vi "STM_Client.vi"() -> ()   [LabVIEW 2019, in "RemoteControl.STM.lvclass"]
uses:
  RemoteControl.STM.lvclass
  <vilib>/NI/STM/SubVIs/MetaDataElement.ctl
  <vilib>/NI/STM/TCP/Read Meta Data (TCP Ref).vi
  <vilib>/NI/STM/TCP/Get Connection Reference (TCP).vi
  <vilib>/NI/STM/TCP/Read Meta Data (TCP Clst).vi
  <userlib>/_OpenG.lib/numeric/numeric.llb/Random Number Within Range - I32__ogtk.vi
  <vilib>/NI/STM/TCP/Write Message (TCP).vi
  <vilib>/NI/STM/TCP/Read Message (TCP).vi
  <userlib>/_OpenG.lib/error/error.llb/Filter Error Codes (Array)__ogtk.vi
  <vilib>/NI/STM/NI STM.lvlib
panel:
  out "Numeric 2":i32
  out "Numeric":i32
  out "messsages/s":dbl
  in  "stop":bool
  out "reponse command":string
  out "response data":string
  out "Command":string
  out "duration ms":u32
  in  "remote address":string
  out "meta data\n(available commands)":T1[](array[typedef])
  out "error out":errorcluster
  # "CLIENT (API)"
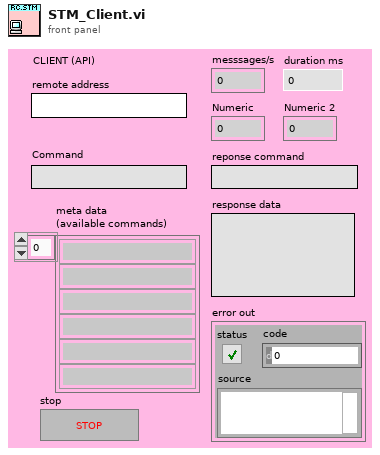
[diagram p1: front panel]
types:
  T1 = typedef "NI STM.lvlib/MetaDataElement.ctl" = string
  T2 = typedef "NI STM.lvlib/TCP Connection Info.ctl" = cluster{"connection ID":refnum<k5>, "meta data":T1[]}
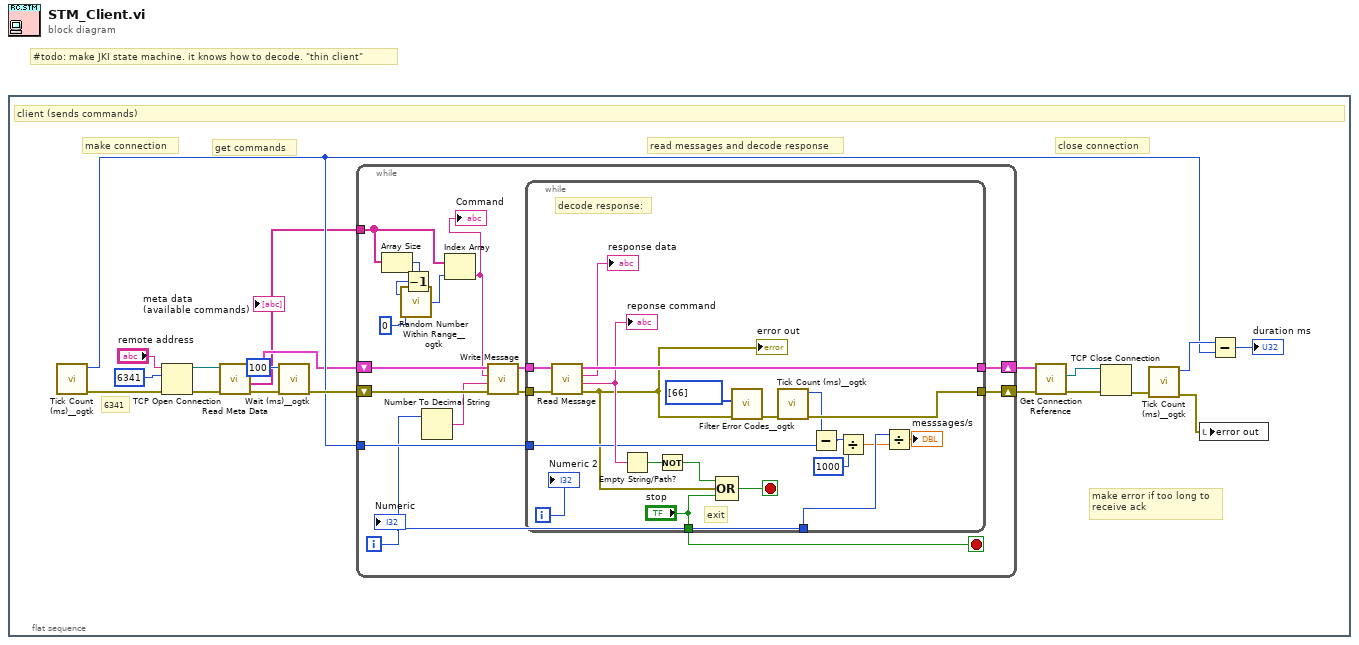
[diagram p0: block diagram]
diagram:
  # "#todo: make JKI state machine. it knows how to decode. \"thin client\""
  n1 = flat-sequence {
    frame #0 {
      # "close connection"
      # "read messages and decode response"
      # "get commands"
      # "make connection"
      # "6341"
      # "make error if too long to\nreceive ack"
      # "client (sends commands)"
      n2 = call <userlib>:"Tick Count (ms)__ogtk.vi"() -> ("error out"=w14:errorcluster, "millisecond timer value"=w4:u32)  [unwired: 10 in]
      n3 = TCP Open Connection(address="remote address", remote port or service name=u16 6341, error in (no error)=w14) -> (connection ID=w18:refnum<k5>, error out=w19:errorcluster)  [unwired: 2 in]
      n4 = call-poly <vilib>:"Read Meta Data.vi"("error in"=w19, "connection ID"=w18) -> ("error out"=w7:errorcluster, "meta data"=w2:T1[], "connection info out"=w3:T2)  [unwired: 7 in]
      "meta data\n(available commands)" <- w2
      n5 = call <userlib>:"Wait (ms)__ogtk.vi"("error in (no error)"=w7, "milliseconds to wait"=u32 100) -> ("error out"=w6:errorcluster)  [unwired: 8 in, 1 out]
      n6 = while {
        shift-right: [w33] -> w13
        shift-left: w6 -> [w28]
        shift-right: [w32] -> w12
        shift-left: w3 -> [w31]
        tunnel: w4 -> [w29]
        tunnel: w2 -> [w25]
        i -> [w21]
        stop <- w30 stop-if-true
        n7 = Array Size(array=w25) -> (size(s)=w26:i32)
        n8 = Decrement(x=w26) -> (x-1=w22:i32)
        n9 = call-poly <userlib>:"Random Number Within Range__ogtk.vi"("High"=w22, "Low"=0) -> ("Random Number"=w23:i32)  [unwired: 3 in]
        n10 = Number To Decimal String(number=w21) -> (decimal integer string=w20:string)  [unwired: 1 in]
        n11 = Index Array(array=w25, index=w23) -> (element=w24:T1)
        "Command" <- w24
        n12 = call-poly <vilib>:"Write Message.vi"("error in"=w28, "data"=w20, "name"=w24, "connection info in"=w31) -> ("error out"=w35:errorcluster, "connection info out"=w34:T2)  [unwired: 6 in]
        n13 = while {
          tunnel: w35 -> [w56]
          tunnel: w34 -> [w55]
          tunnel: [w45] -> w33
          tunnel: [w54] -> w32
          tunnel: ["stop"] -> w30
          tunnel: w29 -> [w43]
          tunnel: w21 -> [w40]
          i -> [w37]
          stop <- w53 stop-if-true
          # "decode response:"
          # "exit"
          n14 = call-poly <vilib>:"Read Message.vi"("error in"=w56, "connection info in"=w55) -> ("error out"=w36:errorcluster, "name"=w50:T1, "data string"=→"response data":string, "connection info out"=w54:T2)  [unwired: 2 in, 4 out]
          "reponse command" <- w50
          "error out" <- w36
          n15 = Empty String/Path?(string/path=w50) -> (empty?=w49:bool)
          n16 = Not(x=w49) -> (.not. x?=w48:bool)
          n17 = Compound Arithmetic op=OR(w48, w36, "stop") -> (w53:bool)
          n18 = call-poly <userlib>:"Filter Error Codes__ogtk.vi"("Error In"=w36, "Error Codes to Filter"=i32[] [66]) -> ("Error Out"=w46:errorcluster)  [unwired: 7 in, 2 out]
          n19 = call <userlib>:"Tick Count (ms)__ogtk.vi"("error in (no error)"=w46) -> ("error out"=w45:errorcluster, "millisecond timer value"=w44:u32)  [unwired: 9 in]
          n20 = Subtract(x=w44, y=w43) -> (x-y=w42:u32)
          n21 = Divide(x=w42, y=u32 1000) -> (x/y=w39:dbl)
          n22 = Divide(x=w40, y=w39) -> (x/y=→"messsages/s":dbl)
          "Numeric 2" <- w37
        }
        "Numeric" <- w21
      }
      n23 = call-poly <vilib>:"Get Connection Reference.vi"("error in"=w13, "connection info in"=w12) -> ("error out"=w16:errorcluster, "connection ID out"=w15:refnum<k5>)  [unwired: 7 in, 1 out]
      n24 = TCP Close Connection(connection ID=w15, error in (no error)=w16) -> (error out=w11:errorcluster)  [unwired: 1 in, 1 out]
      n25 = call <userlib>:"Tick Count (ms)__ogtk.vi"("error in (no error)"=w11) -> ("error out"=w1:errorcluster, "millisecond timer value"=w9:u32)  [unwired: 9 in]
      n26 = local write "error out"(w1) -> ()
      n27 = Subtract(x=w9, y=w4) -> (x-y=→"duration ms":u32)
    }
  }
